vi "Which Affected Item Clicked.vi"(10 "User VI Ref":refnum<vi>, 11 "Affected Items":T2) -> (0 "Compiled Affected Items":T1[](array[typedef]), 1 "Affected Item Enum Dummy":T1=enum."Named Un/Bundler", 3 "Affected Items Out":T2)   [LabVIEW 2023]
doc: "Wires are checked for having a data type of a cluster\n\nTerminal looks for a terminal on a named bundler or unbunder\n\nWe differentiate between terminals that are controls and indicators, and those that are cluster types on other nodes (SubVIs, etc).\n\nCluster Terminal Count is the number of cluster control and indicator terminals selected, OR the number of input/output terminals displayed on a bundle/unbundle by name.\n\nAffected Item can fall under more than on category, and we will want menu items for each relevent category. Therefore, the affected items enum is output as an array."
uses:
  BundleMagic.ctl
  controls/Affected Item Enum.ctl
panel:
  # "Dummy  for BD function"
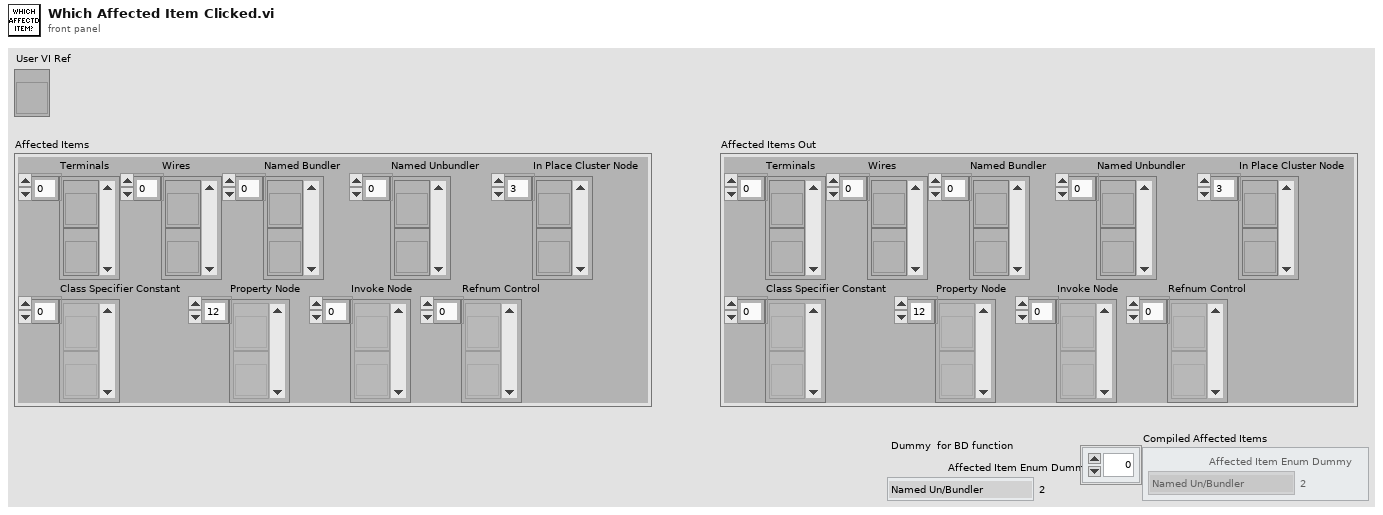
[diagram p1: front panel]
types:
  T1 = typedef "Affected Item Enum.ctl" = enum16{"[NONE]", "Cluster Wire", "Named Un/Bundler", "In Place", "Cluster Terminal", "Reference Wire", "Reference Terminal", "Property Node", "Class Specifier Constant", "Invoke Node", "Refnum Control"}
  T2 = typedef "BundleMagic.ctl" = cluster{"Terminals":refnum<vi>[], "Wires":refnum<vi>[], "Named Bundler":refnum<vi>[], "Named Unbundler":refnum<vi>[], "In Place Cluster Node":refnum<vi>[], "Class Specifier Constant":refnum<vi>[], "Property Node":refnum<vi>[], "Invoke Node":refnum<vi>[], "Refnum Control":refnum<vi>[]}
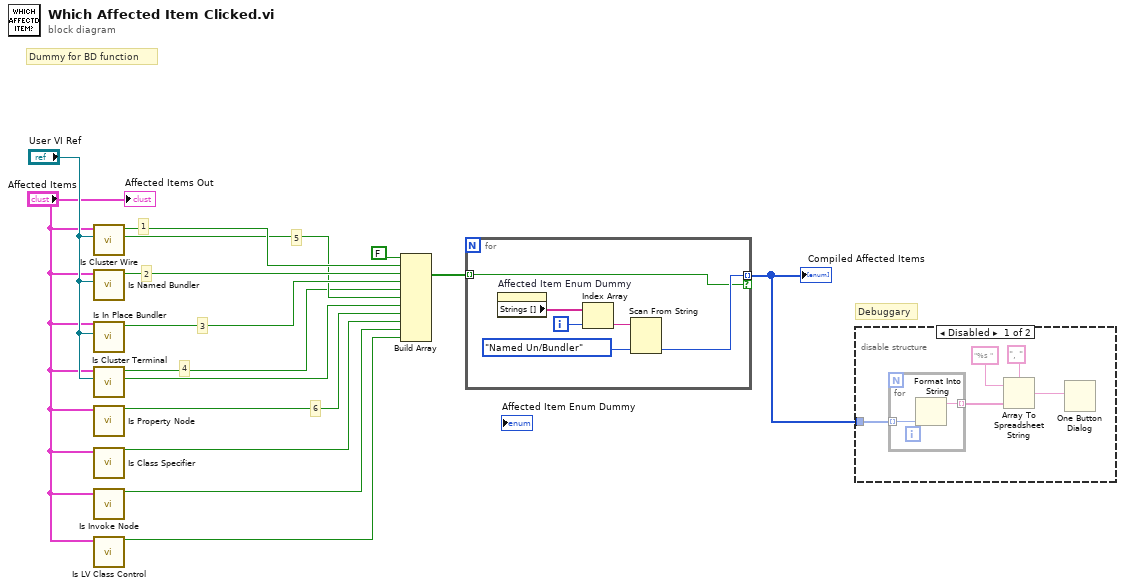
[diagram p0: block diagram]
diagram:
  # "5"
  # "Debuggary"
  # "Dummy for BD function"
  # "6"
  # "4"
  # "3"
  # "2"
  # "1"
  n1 = call "Is Cluster Wire.vi"("User VI Ref"="User VI Ref", "Affected Items"="Affected Items") -> ("Refnum Wire?"=w10:bool, "Cluster Wire?"=w15:bool)  [unwired: 6 in, 2 out]
  n2 = call "Is Named Bundler.vi"("User VI Ref"="User VI Ref", "Affected Items"="Affected Items") -> ("Named Cluster Un/bundle Selected"=w13:bool)  [unwired: 3 in, 6 out]
  n3 = call "Is In Place Bundler.vi"("User VI Ref"="User VI Ref", "Affected Items"="Affected Items") -> ("In Place Bundler Selected"=w12:bool)  [unwired: 6 in, 3 out]
  n4 = call "Is Cluster Terminal.vi"("User VI Ref"="User VI Ref", "Affected Items"="Affected Items") -> ("Refnum Term?"=w9:bool, "Cluster Term?"=w1:bool)  [unwired: 7 in, 1 out]
  n5 = call "Is Property Node.vi"("Affected Items"="Affected Items") -> ("Property Node?"=w8:bool)  [unwired: 10 in]
  n6 = call "Is Class Specifier.vi"("Affected Items"="Affected Items") -> ("Class Specifier Constant?"=w7:bool)  [unwired: 10 in]
  n7 = call "Is Invoke Node.vi"("Affected Items"="Affected Items") -> ("Invoke Node?"=w5:bool)  [unwired: 10 in]
  n8 = call "Is LV Class Control.vi"("Affected Items"="Affected Items") -> ("Refnum?"=w4:bool)  [unwired: 10 in]
  n9 = Build Array(FALSE, w15, w13, w12, w1, w10, w9, w8, w7, w5, w4) -> (w6:bool[])
  n10 = for {
    tunnel: w6 -> [w18] mode=indexing
    tunnel: [w21] -> w3 mode=indexing if=w18
    i -> [w19]
    n11 = property on="Affected Item Enum Dummy" class="Enum (strict)"() -> ("Strings []"=w17:string[])  [unwired: 2 in, 2 out]
    n12 = Index Array(array=w17, index=w19) -> (element=w20:string)
    n13 = Scan From String(input string=w20, default 1=Affected_Item_Enum."Named Un/Bundler" ("Affected Item Enum Dummy")) -> (output 1=w21:T1)  [unwired: 3 in, 3 out]
  }
  "Compiled Affected Items" <- w3
  n14 = disable-structure shown="Disabled" {
    disable-tunnel: w3 -> [w26 _]
    frame Disabled {
      n15 = for {
        tunnel: w26 -> [w28] mode=indexing
        tunnel: [w27] -> w25 mode=indexing
        n16 = Format Into String(w28) -> (resulting string=w27:string)  [unwired: 3 in, 1 out]
      }
      n17 = Array To Spreadsheet String(delimiter (Tab)=", ", array=w25, 3:"%s " ("delimiter (Tab)")) -> (spreadsheet string=w22:string)
      n18 = One Button Dialog(message=w22) -> ()  [unwired: 1 in, 1 out]
    }
    frame Enabled {
    }
  }
  "Affected Items Out" <- "Affected Items"
